vi "is_h5.vi"(1 "path":path) -> (0 "is h5?":bool)   [LabVIEW 2015]
uses:
  <userlib>/_OpenG.lib/file/file.llb/Valid Path - Traditional__ogtk.vi
  <userlib>/_OpenG.lib/file/file.llb/Strip Path Extension - Path__ogtk.vi
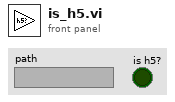
[diagram p1: front panel]
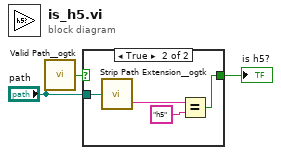
[diagram p0: block diagram]
diagram:
  n1 = call-poly <userlib>:"Valid Path__ogtk.vi"("path"="path") -> ("valid"=w3:bool)
  n2 = case shown="True" w3 {
    selector: w3 -> [w4 _]
    tunnel: "path" -> [_ w8]
    tunnel: [w4 w5] -> w1
    frame False {
    }
    frame True {
      n3 = call-poly <userlib>:"Strip Path Extension__ogtk.vi"("path"=w8) -> ("extension"=w7:string)  [unwired: 1 out]
      n4 = Equal?(x=w7, y="h5") -> (x = y?=w5:bool)
    }
  }
  "is h5?" <- w1
